vi "SetupSystemSection.vi"(8 "error in (no error)":errorcluster, 11 "Node Ptr":u64 format="%.0x") -> (0 "error out":errorcluster, 1 "Error Code Ref":T1 format="%.0x", 2 "Triggered Ref":T1 format="%.0x", 3 "Parent Ref Out":T1 format="%.0x", 4 "Trigger Ref":T1 format="%.0x", 5 "Logging Ref":T1 format="%.0x")   [LabVIEW 2024, in "Embedded TDMS Logger System Explorer.lvlib"]
doc: "Creates the system group and system channels for the Custom Device:\n- The trigger channel (input)\n- The trigger/logging status channel (output)\n- The error code channel (output)\n\nNamed under the Logging & Diagnostics system group."
uses:
  Embedded TDMS Logger System Explorer.lvlib
  <vilib>/NI VeriStand/Custom Device API/Custom Device Item Ref.ctl
  <vilib>/NI VeriStand/Custom Device API/Custom Device Channel.ctl
  <vilib>/NI VeriStand/Custom Device API/Custom Device Channel Type.ctl
  Shared/Constants.vi
  <vilib>/NI VeriStand/Custom Device API/Custom Device API.lvlib
  Shared/Embedded TDMS Logger Shared.lvlib
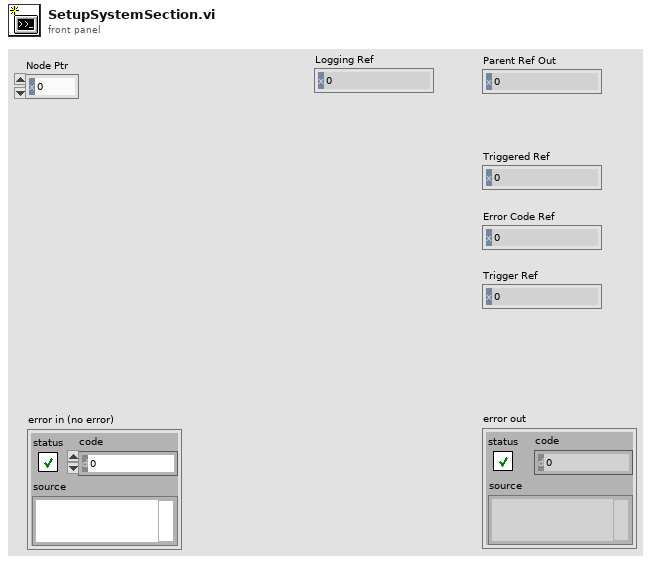
[diagram p1: front panel]
types:
  T1 = typedef "Custom Device API.lvlib/Custom Device Item Ref.ctl" = u64
  T2 = typedef "Custom Device API.lvlib/Custom Device Channel.ctl" = cluster{"Type":T3, "Units":string, "Default Value":dbl, "Faultable":bool, "Scalable":bool}
  T3 = typedef "Custom Device API.lvlib/Custom Device Channel Type.ctl" = enum16{"Input", "Output"}
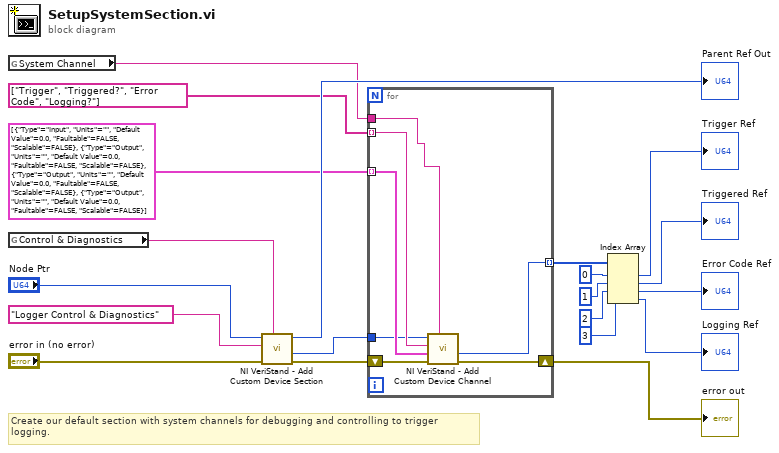
[diagram p0: block diagram]
diagram:
  # "Create our default section with system channels for debugging and controlling to trigger\nlogging."
  n1 = global read "Constants.vi" "System Channel"() -> (w3:string)
  n2 = global read "Constants.vi" "Control & Diagnostics"() -> (w17:string)
  n3 = call <vilib>:"NI VeriStand - Add Custom Device Section.vi"("GUID (Default Section)"=w17, "error in (no error)"="error in (no error)", "Section Name"="Logger Control & Diagnostics", "Parent Ref in"="Node Ptr") -> ("error out"=w4:errorcluster, "Section Ptr"=w9:T1, "Parent Ref out"=→"Parent Ref Out":T1)  [unwired: 4 in, 1 out]
  n4 = for {
    tunnel: [w23] -> w12 mode=indexing
    tunnel: string[] ["Trigger", "Triggered?", "Error Code", "Logging?"] -> [w27] mode=indexing
    tunnel: T2[] [{"Type"=enum."Input", "Units"="", "Default Value"=0.0, "Faultable"=FALSE, "Scalable"=FALSE}, {"Type"=enum."Output", "Units"="", "Default Value"=0.0, "Faultable"=FALSE, "Scalable"=FALSE}, {"Type"=enum."Output", "Units"="", "Default Value"=0.0, "Faultable"=FALSE, "Scalable"=FALSE}, {"Type"=enum."Output", "Units"="", "Default Value"=0.0, "Faultable"=FALSE, "Scalable"=FALSE}] -> [w26] mode=indexing
    shift-right: [w24] -> w5
    shift-left: w4 -> [w25]
    tunnel: w9 -> [w22]
    tunnel: w3 -> [w21]
    n5 = call <vilib>:"NI VeriStand - Add Custom Device Channel.vi"("GUID (Default Channel)"=w21, "error in (no error)"=w25, "Channel"=w26, "Channel Name"=w27, "Parent Ref in"=w22) -> ("error out"=w24:errorcluster, "Channel Ref"=w23:T1)  [unwired: 3 in, 2 out]
  }
  "error out" <- w5
  n6 = Index Array(array=w12, index #1=0 ("index"), index #2=1 ("index"), index #3=2 ("index"), index #4=3 ("index")) -> (element #1=→"Trigger Ref":T1, element #2=→"Triggered Ref":T1, element #3=→"Error Code Ref":T1, element #4=→"Logging Ref":T1)
